vi "Actor Setup.vi"(10 "Actor":refnum<class "Actor.lvclass">, 11 "Dev Actor in":refnum<class "Dev Actor.lvclass">) -> (0 "error out":errorcluster, 3 "Dev Actor out":refnum<class "Dev Actor.lvclass">)   [LabVIEW 2021, in "Dev Actor.lvlib" / "Dev Actor.lvclass"]
uses:
  Dev Actor.lvclass
  LVCAM/LVCAM/Actor/Actor.lvclass
  ABD Panel/ABD Panel.lvclass
  C:/PPLs/LabVIEW-Composed-Actor-Model-LVCAM/LabVIEW-Composed-Actor-Model-LVCAM/Panel/Panel.lvclass
  Dev Actor.lvclass/Dev Actor.ctl
  Panel/Panel.lvclass
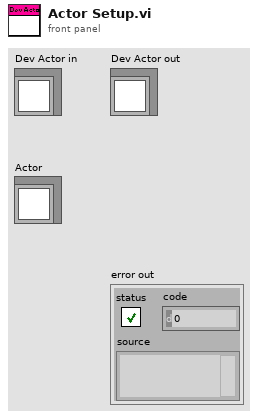
[diagram p1: front panel]
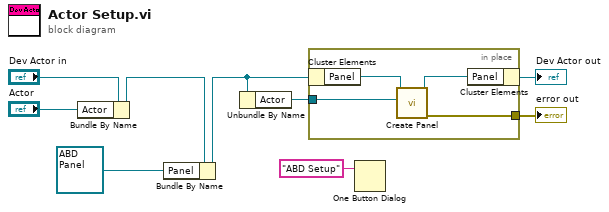
[diagram p0: block diagram]
diagram:
  n1 = Bundle By Name(cluster="Dev Actor in", "Actor"="Actor") -> (w4:refnum<class "Dev Actor.lvclass">)
  n2 = Bundle By Name(cluster=w4, "Panel"=refnum<class "ABD Panel.lvclass"> refnum ("ABD Panel.lvclass")) -> (w2:refnum<class "Dev Actor.lvclass">)
  n3 = Unbundle By Name(w2) -> ("Actor"=w3:refnum<class "Actor.lvclass">)
  n4 = in-place {
    in-place-border: [w11] -> w5
    in-place-border: w3 -> [w10]
    n5 = in-place-cluster #1(w2) -> ("Panel"=w13:refnum<class "Panel.lvclass">)
    n6 = call "Create Panel.vi"("Actor"=w10, "Panel in"=w13) -> ("error out"=w11:errorcluster, "Panel out"=w12:refnum<class "Panel.lvclass">)  [unwired: 8 in]
    n7 = in-place-cluster #1("Panel"=w12) -> (→"Dev Actor out":refnum<class "Dev Actor.lvclass">)
  }
  "error out" <- w5
  n8 = One Button Dialog(message="ABD Setup") -> ()  [unwired: 1 in, 1 out]
